vi "ecg to wave.vi"   [LabVIEW 2014]
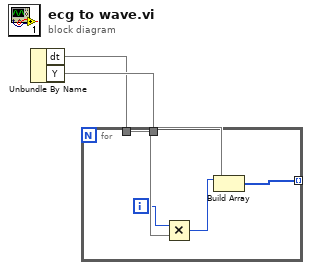
[diagram p0: block diagram]
diagram:
  n1 = Unbundle By Name() -> (w3:waveform(dbl), "dt"=w2, "Y"=w4)
  n2 = for {
    tunnel: w4 -> [w9]
    tunnel: [w8] -> w1 mode=indexing
    tunnel: w2 -> [w7]
    i -> [w6]
    n3 = Multiply(x=w6, y=w7) -> (x*y=w5:i32)
    n4 = Build Array(w5, w9) -> (w8:i32[])
  }
